vi "System Time Display.vi"() -> ()   [LabVIEW 2016]
panel:
  out "PM":bool
  out "AM":bool
  out ".. 2":bool
  out ". 2":bool
  out "S 1":T1
  out "S 2":T1
  out "..":bool
  out ".":bool
  out "M 2":T1
  out "M 1":T1
  out "H 2":T1
  out "H 1":T1
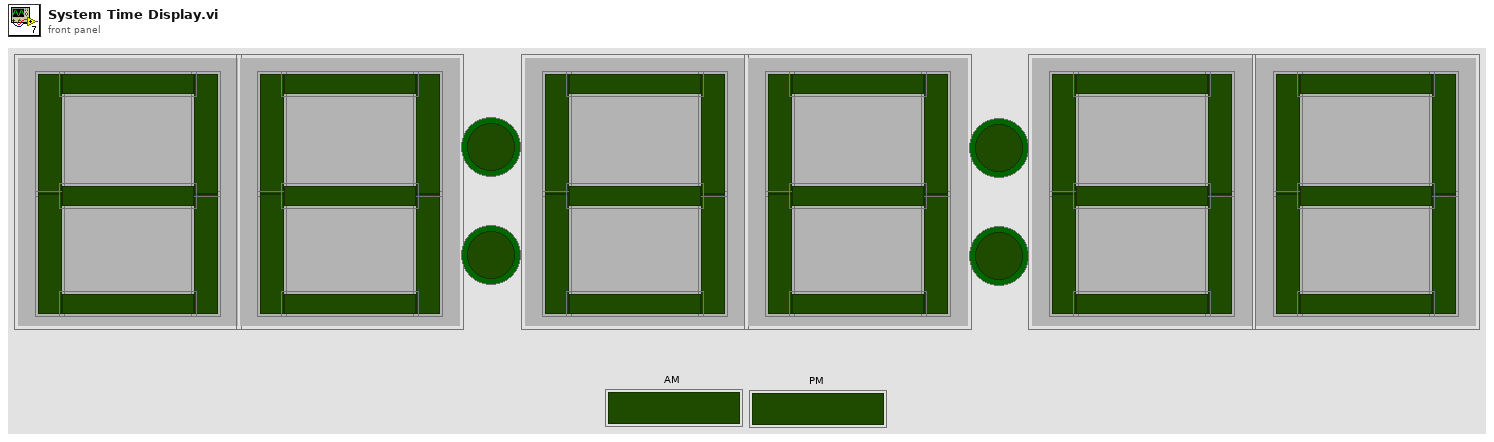
[diagram p1: front panel]
types:
  T1 = cluster{"f":bool, "e":bool, "c":bool, "b":bool, "d":bool, "g":bool, "a":bool}
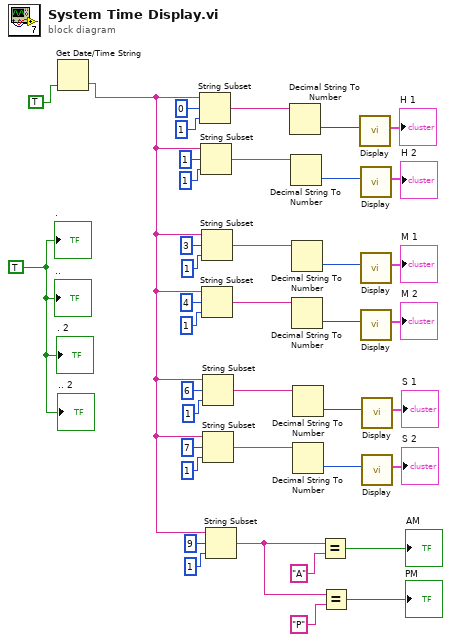
[diagram p0: block diagram]
diagram:
  w9 = TRUE
  n1 = Get Date/Time String(want seconds? (F)=TRUE) -> (time string=w6:string)  [unwired: 2 in, 1 out]
  n2 = String Subset(string=w6, offset (0)=0, length (rest)=1 ("length (rest)")) -> (substring=w38:string)
  n3 = String Subset(string=w6, offset (0)=1, length (rest)=1 ("length (rest)")) -> (substring=w36:string)
  n4 = String Subset(string=w6, offset (0)=3, length (rest)=1 ("length (rest)")) -> (substring=w37:string)
  n5 = String Subset(string=w6, offset (0)=4, length (rest)=1 ("length (rest)")) -> (substring=w28:string)
  n6 = String Subset(string=w6, offset (0)=6, length (rest)=1 ("length (rest)")) -> (substring=w10:string)
  n7 = String Subset(string=w6, offset (0)=7, length (rest)=1 ("length (rest)")) -> (substring=w15:string)
  n8 = String Subset(string=w6, offset (0)=9, length (rest)=1 ("length (rest)")) -> (substring=w3:string)
  n9 = Decimal String To Number(string=w38) -> (number=w39:i32)  [unwired: 2 in, 1 out]
  n10 = Decimal String To Number(string=w36) -> (number=w34:i32)  [unwired: 2 in, 1 out]
  n11 = Decimal String To Number(string=w37) -> (number=w35:i32)  [unwired: 2 in, 1 out]
  n12 = Decimal String To Number(string=w28) -> (number=w29:i32)  [unwired: 2 in, 1 out]
  n13 = Decimal String To Number(string=w10) -> (number=w11:i32)  [unwired: 2 in, 1 out]
  n14 = Decimal String To Number(string=w15) -> (number=w14:i32)  [unwired: 2 in, 1 out]
  n15 = Equal?(x=w3, y="A") -> (x = y?=→"AM":bool)
  n16 = Equal?(x=w3, y="P") -> (x = y?=→"PM":bool)
  n17 = call "Display.vi"("Case Selector"=w39) -> ("Cluster"=→"H 1":T1)  [unwired: 10 in]
  n18 = call "Display.vi"("Case Selector"=w34) -> ("Cluster"=→"H 2":T1)  [unwired: 10 in]
  n19 = call "Display.vi"("Case Selector"=w35) -> ("Cluster"=→"M 1":T1)  [unwired: 10 in]
  n20 = call "Display.vi"("Case Selector"=w29) -> ("Cluster"=→"M 2":T1)  [unwired: 10 in]
  n21 = call "Display.vi"("Case Selector"=w11) -> ("Cluster"=→"S 1":T1)  [unwired: 10 in]
  n22 = call "Display.vi"("Case Selector"=w14) -> ("Cluster"=→"S 2":T1)  [unwired: 10 in]
  "." <- w9
  ".." <- w9
  ". 2" <- w9
  ".. 2" <- w9
